vi "CHECK arm geometry.vi"(9 "select limit":u16(ring) items=["typical", "HANGAR"], 11 "arm angle (deg)":dbl(knob) min=-30.0 max=30.0 scale=30.0..-30.0) -> (1 "arm shuttle":cluster{"x":dbl, "y":dbl}={"x"=-9.11895003862225, "y"=13.0}, 3 "stroke max":dbl=17.75)   [LabVIEW 2020]
panel:
  out "angle (PI)":dbl=0.5 format="%.3g"
  out "In Range?":bool
  out "link to arm":cluster{"x":dbl, "y":dbl}={"x"=2.5000000000000004, "y"=16.0}
  out "hook ctr wrt CG":cluster{"x":dbl, "y":dbl}={"x"=4.000000000000003, "y"=46.25}
  in  "robot frame length (in)":dbl=30.0 format="%#_13g"
  in  "testing?":bool
  in  "hook outer diam (in)":dbl=4.0 format="%.3g"
  in  "coords to link (in)":cluster{"x":dbl, "y":dbl}[](array[cluster])=[{"x"=0.0, "y"=9.0}, {"x"=1.5, "y"=0.0}]
  in  "screw link (in)":dbl=12.0 format="%.3g"
  in  "stop":bool
  out "XY Graph":cluster{dbl[], dbl[]}[](graph)=[{[-31.0, -31.0, 31.0, 31.0], [0.0, 66.0, 66.0, 0.0]}, {[-29.0, -29.0, 29.0, 29.0], [0.0, 64.0, 64.0, 0.0]}, {[4.0, 4.000000000000003], [7.0, 46.25]}, {[2.5000000000000004, -9.11895003862225], [16.0, 13.0]}]
  in  "arm coords (in)":cluster{"x":dbl, "y":dbl}[](array[cluster])=[{"x"=0.0, "y"=32.5}, {"x"=0.0, "y"=3.0}, {"x"=0.0, "y"=3.75}]
  in  "screw pin AG (in)":dbl=13.0 format="%.3g"
  in  "shoulder pin back from CG (in)":dbl=4.0 format="%.3g"
  in  "shoulder pin AG (in)":dbl=7.0 format="%.3g"
  in  "Stroke (in)":dbl(slide) scale=0.0..24.0
  out "height limit (in)":dbl=66.0 format="%.3g"
  in  "frame reach limit (in)":dbl=16.0 format="%.3g"
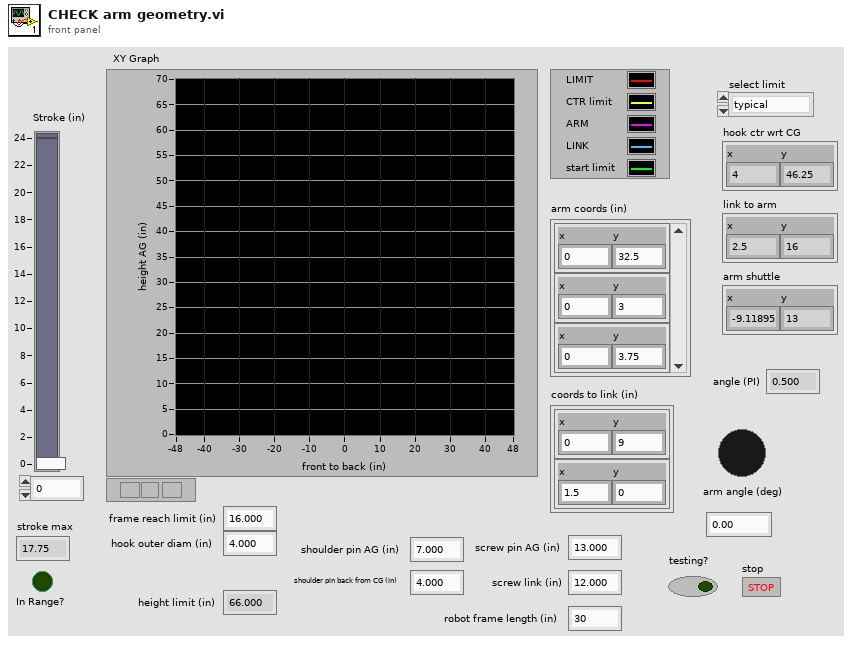
[diagram p1: front panel]
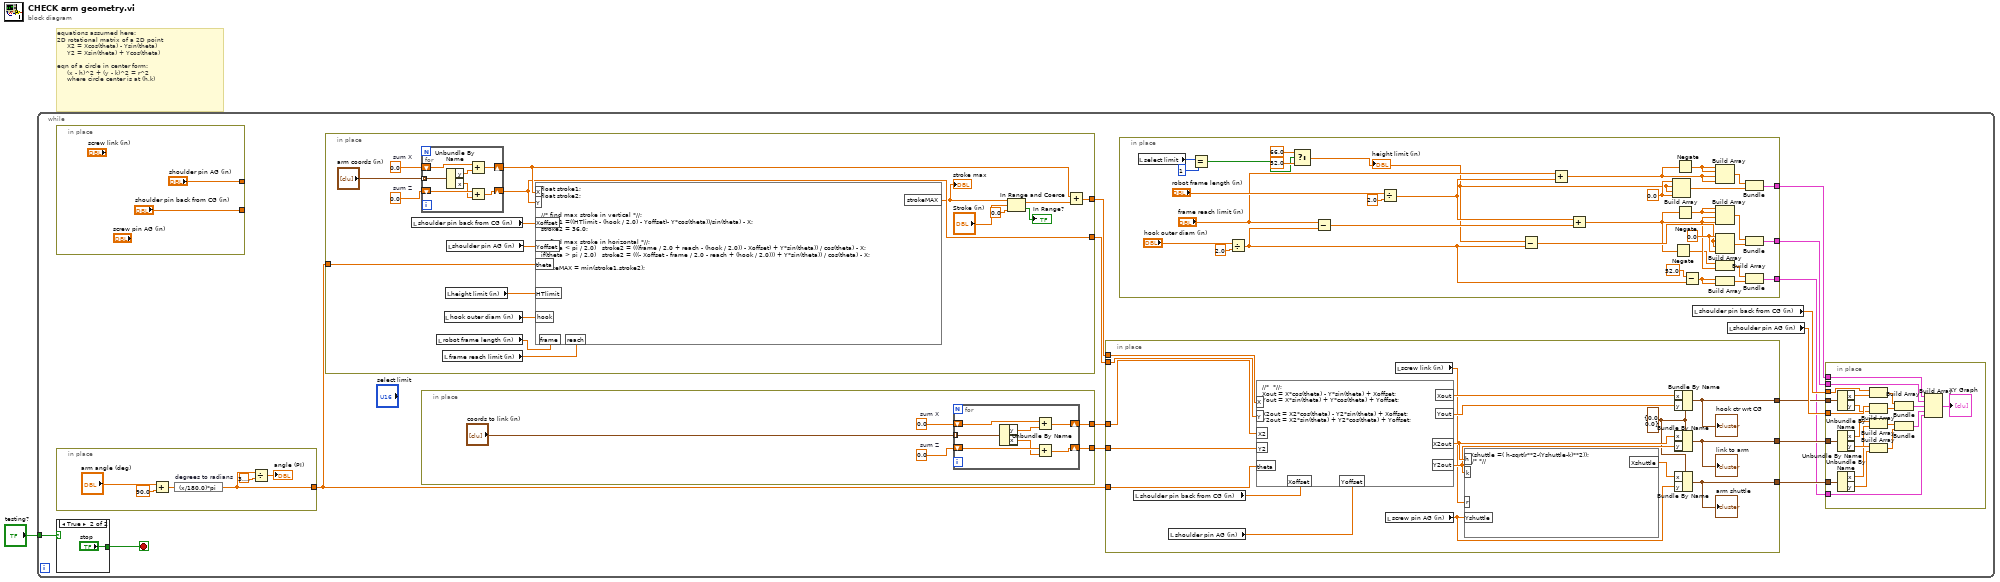
[diagram p0: block diagram]
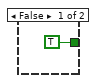
[diagram p2: hidden frame]
diagram:
  # "equations assumed here:\n2D rotational matrix of a 2D point\n     X2 = Xcos(theta) - Ysin(theta)\n     Y2 = Xsin(theta) + Ycos(theta)\n\neqn of a circle in center form:\n     (x - h)^2 + (y - k)^2 = r^2\n     where circle center is at (h,k)"
  n1 = while {
    tunnel: "testing?" -> [w14]
    stop <- w16 stop-if-true
    n2 = in-place {
      in-place-border: ["shoulder pin back from CG (in)"] -> _
      in-place-border: ["shoulder pin AG (in)"] -> _
    }
    n3 = in-place {
      in-place-border: [w43] -> w3
      n4 = Add(x="arm angle (deg)", y=90.0) -> (x+y=w40:dbl)
      n5 = expression code="(x/180.0)*pi" "degrees to radians"(w40) -> (w43:dbl)
      n6 = Divide(x=w43, y=3.141592653589793) -> (x/y=→"angle (PI)":dbl)
    }
    n7 = case shown="True" w14 {
      tunnel: [TRUE ("stop") "stop"] -> w16
      frame False {
      }
      frame True {
      }
    }
    n8 = in-place {
      in-place-border: [w124] -> w11
      in-place-border: [w118] -> w10
      in-place-border: w3 -> [w116]
      w127 = 0.0  # sum X
      w126 = 0.0  # sum Z
      n9 = local read "shoulder pin back from CG (in)"() -> (w121:dbl)
      n10 = for {
        tunnel: "arm coords (in)" -> [w135] mode=indexing
        shift-right: [w133] -> w118
        shift-left: w126 -> [w134]
        shift-right: [w132] -> w119
        shift-left: w127 -> [w131]
        n11 = Unbundle By Name(w135) -> ("y"=w130:dbl, "x"=w129:dbl)
        n12 = Add(x=w131, y=w130) -> (x+y=w132:dbl)
        n13 = Add(x=w134, y=w129) -> (x+y=w133:dbl)
      }
      n14 = local read "robot frame length (in)"() -> (w111:dbl)
      n15 = local read "frame reach limit (in)"() -> (w112:dbl)
      n16 = local read "hook outer diam (in)"() -> (w114:dbl)
      n17 = local read "height limit (in)"() -> (w115:dbl)
      n18 = local read "shoulder pin AG (in)"() -> (w120:dbl)
      n19 = formula code="float stroke1;\nfloat stroke2;\n\n\n//* find max stroke in vertical *//;\nstroke1 =((HTlimit - (hook / 2.0) - Yoffset)- Y*cos(theta))/sin(theta) - X;\nstroke2 = 36.0;\n\n//* find max stroke in horizontal *//;\nif(theta < pi / 2.0)   stroke2 = (((frame / 2.0 + reach - (hook / 2.0)) - Xoffset) + Y*sin(theta)) / cos(theta) - X;\nif(theta > pi / 2.0)   stroke2 = (((- Xoffset - frame / 2.0 - reach + (hook / 2.0))) + Y*sin(theta)) / cos(theta) - X;\n\nstrokeMAX = min(stroke1,stroke2);"("Xoffset"=w121, "Yoffset"=w120, "theta"=w116, "X"=w119, "Y"=w118, "HTlimit"=w115, "hook"=w114, "frame"=w111, "reach"=w112) -> ("strokeMAX"=w117:dbl)
      "stroke max" <- w117
      n20 = In Range and Coerce(upper limit=w117, x="Stroke (in)", lower limit=0.0) -> (coerced(x)=w123:dbl, In Range?=→"In Range?":bool)
      n21 = Add(x=w119, y=w123) -> (x+y=w124:dbl)
    }
    n22 = in-place {
      in-place-border: [w66] -> w12
      in-place-border: [w64] -> w13
      w68 = 0.0  # sum X
      w67 = 0.0  # sum Z
      n23 = for {
        tunnel: "coords to link (in)" -> [w75] mode=indexing
        shift-right: [w73] -> w66
        shift-left: w67 -> [w74]
        shift-right: [w72] -> w64
        shift-left: w68 -> [w71]
        n24 = Unbundle By Name(w75) -> ("y"=w70:dbl, "x"=w69:dbl)
        n25 = Add(x=w71, y=w70) -> (x+y=w72:dbl)
        n26 = Add(x=w74, y=w69) -> (x+y=w73:dbl)
      }
    }
    n27 = in-place {
      in-place-border: w3 -> [w61]
      in-place-border: w13 -> [w58]
      in-place-border: w12 -> [w57]
      in-place-border: w11 -> [w56]
      in-place-border: w10 -> [w55]
      in-place-border: [w46] -> w7
      in-place-border: [w45] -> w6
      in-place-border: [w44] -> w5
      w47 = cluster{"x":dbl, "y":dbl} {"x"=0.0, "y"=0.0} ("Cluster")
      n28 = local read "shoulder pin back from CG (in)"() -> (w54:dbl)
      n29 = local read "shoulder pin AG (in)"() -> (w53:dbl)
      n30 = formula code="//*  *//;\nXout = X*cos(theta) - Y*sin(theta) + Xoffset;\nYout = X*sin(theta) + Y*cos(theta) + Yoffset;\n\nX2out = X2*cos(theta) - Y2*sin(theta) + Xoffset;\nY2out = X2*sin(theta) + Y2*cos(theta) + Yoffset;"("X"=w56, "Y"=w55, "theta"=w61, "X2"=w58, "Y2"=w57, "Xoffset"=w54, "Yoffset"=w53) -> ("Xout"=w60:dbl, "Yout"=w59:dbl, "X2out"=w52:dbl, "Y2out"=w51:dbl)
      n31 = local read "screw pin AG (in)"() -> (w48:dbl)
      n32 = local read "screw link (in)"() -> (w50:dbl)
      n33 = formula code="Xshuttle =( h-sqrt(r**2-(Yshuttle-k)**2));\n//* *//"("h"=w52, "k"=w51, "Yshuttle"=w48, "r"=w50) -> ("Xshuttle"=w49:dbl)
      n34 = Bundle By Name(cluster=w47, "x"=w60, "y"=w59) -> (w44:cluster{"x":dbl, "y":dbl})
      "hook ctr wrt CG" <- w44
      n35 = Bundle By Name(cluster=w47, "x"=w52, "y"=w51) -> (w45:cluster{"x":dbl, "y":dbl})
      "link to arm" <- w45
      n36 = Bundle By Name(cluster=w47, "x"=w49, "y"=w48) -> (w46:cluster{"x":dbl, "y":dbl})
      "arm shuttle" <- w46
    }
    n37 = in-place {
      in-place-border: [w102] -> w15
      in-place-border: [w90] -> w4
      in-place-border: [w87] -> w2
      w91 = 0.0 ("element")
      w103 = 0.0 ("element")
      n38 = local read "select limit"() -> (w78:u16)
      n39 = Equal?(x=w78, y=u16 1) -> (x = y?=w76:bool)
      n40 = Divide(x="hook outer diam (in)", y=2.0) -> (x/y=w82:dbl)
      n41 = Select(t=66.0, s=w76, f=52.0) -> (s? t:f=w81:dbl)
      "height limit (in)" <- w81
      n42 = Subtract(x="frame reach limit (in)", y=w82) -> (x-y=w101:dbl)
      n43 = Divide(x="robot frame length (in)", y=2.0) -> (x/y=w95:dbl)
      n44 = Subtract(x=w81, y=w82) -> (x-y=w98:dbl)
      n45 = Add(x="frame reach limit (in)", y=w95) -> (x+y=w93:dbl)
      n46 = Add(x=w95, y=w101) -> (x+y=w86:dbl)
      n47 = Build Array(w91, w81, w81, w91) -> (w97:dbl[])
      n48 = Negate(x=w86) -> (-x=w85:dbl)
      n49 = Negate(x=w93) -> (-x=w92:dbl)
      n50 = Negate(x=w86) -> (-x=w104:dbl)
      n51 = Subtract(x=52.0, y=w82) -> (x-y=w83:dbl)
      n52 = Build Array(w92, w92, w93, w93) -> (w96:dbl[])
      n53 = Build Array(w104, w104, w86, w86) -> (w107:dbl[])
      n54 = Build Array(w103, w98, w98, w103) -> (w108:dbl[])
      n55 = Build Array(w85, w86) -> (w88:dbl[])
      n56 = Build Array(w83, w83) -> (w89:dbl[])
      n57 = Bundle(w96, w97) -> (w90:cluster{dbl[], dbl[]})  [unwired: 1 in]
      n58 = Bundle(w107, w108) -> (w102:cluster{dbl[], dbl[]})  [unwired: 1 in]
      n59 = Bundle(w88, w89) -> (w87:cluster{dbl[], dbl[]})  [unwired: 1 in]
    }
    n60 = local read "shoulder pin back from CG (in)"() -> (w8:dbl)
    n61 = local read "shoulder pin AG (in)"() -> (w9:dbl)
    n62 = in-place {
      in-place-border: w15 -> [w33]
      in-place-border: w8 -> [w29]
      in-place-border: w9 -> [w28]
      in-place-border: w7 -> [w24]
      in-place-border: w6 -> [w27]
      in-place-border: w5 -> [w21]
      in-place-border: w4 -> [w18]
      in-place-border: w2 -> [w17]
      n63 = Unbundle By Name(w21) -> ("x"=w20:dbl, "y"=w19:dbl)
      n64 = Unbundle By Name(w27) -> ("x"=w26:dbl, "y"=w25:dbl)
      n65 = Unbundle By Name(w24) -> ("x"=w22:dbl, "y"=w23:dbl)
      n66 = Build Array(w29, w20) -> (w36:dbl[])
      n67 = Build Array(w28, w19) -> (w37:dbl[])
      n68 = Build Array(w26, w22) -> (w31:dbl[])
      n69 = Build Array(w25, w23) -> (w32:dbl[])
      n70 = Bundle(w36, w37) -> (w34:cluster{dbl[], dbl[]})  [unwired: 1 in]
      n71 = Bundle(w31, w32) -> (w30:cluster{dbl[], dbl[]})  [unwired: 1 in]
      n72 = Build Array(w18, w33, w34, w30, w17) -> (→"XY Graph":cluster{dbl[], dbl[]}[])
    }
  }
